vi "SaveJournalGen.vi"(7 "CheminSauv":path=path "C:/Données/Run003" caption="Fichier de Sauvegarde", 8 "error in":errorcluster, 10 "Include Date_Time":bool=TRUE, 11 "Journal Text":string) -> (0 "error out":errorcluster, 3 "chaîne de journal":string)   [LabVIEW 2019]
doc: "Ce Vi sauvegarde les données sous forme de collonnes dans le fichier texte de sauvegarde"
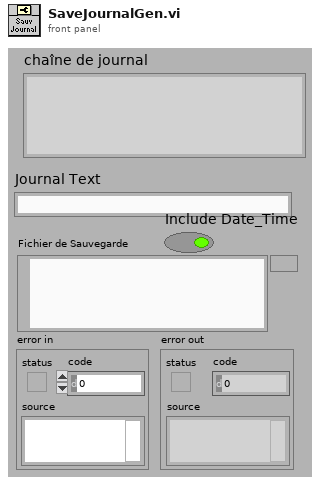
[diagram p1: front panel]
types:
  T1 = enum16{"open", "open or create", "create or replace", "create", "open (read only)"}
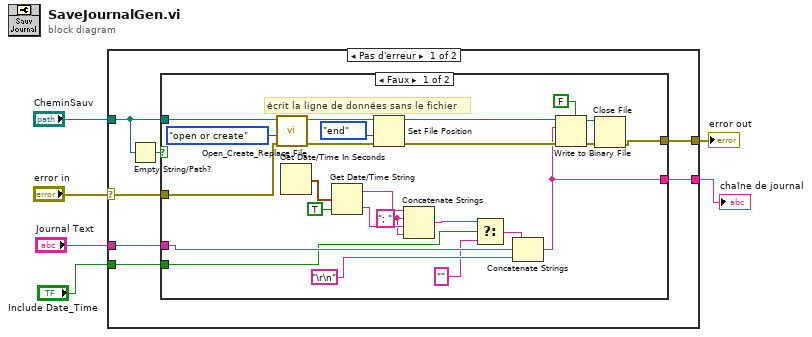
[diagram p0: block diagram]
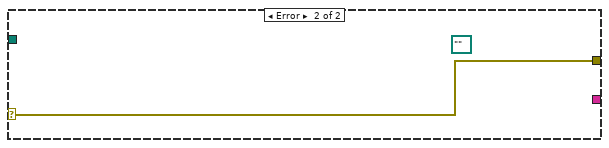
[diagram p3: hidden frame]
diagram:
  n1 = case shown="Pas d'erreur" "error in" {
    selector: "error in" -> [w12 w39]
    tunnel: [w13 w39] -> w6
    tunnel: "CheminSauv" -> [w10 _]
    tunnel: "Journal Text" -> [w9 _]
    tunnel: [w8 _] -> w2
    tunnel: "Include Date_Time" -> [w7 _]
    frame No Error {
      n2 = Empty String/Path?(string/path=w10) -> (empty?=w11:bool)
      n3 = case shown="Faux" w11 {
        tunnel: [w32 w38] -> w13
        tunnel: w12 -> [w31 w38]
        tunnel: w10 -> [w30 _]
        tunnel: w9 -> [w20 _]
        tunnel: [w16 _] -> w8
        tunnel: w7 -> [w14 _]
        frame False {
          w21 = "; " ("élément")
          # "écrit la ligne de données sans le fichier"
          n4 = call <vilib>:"Open_Create_Replace File.vi"("error in (no error)"=w31, "function (open:0)"=T1."open or create", "file path"=w30) -> ("error out"=w37:errorcluster, "refnum"=w33:refnum<file>)  [unwired: 5 in, 2 out]
          n5 = Get Date/Time In Seconds() -> (seconds since 1Jan1904=w23:timestamp)
          n6 = Get Date/Time String(seconds (now)=w23, want seconds? (F)=TRUE ("secondes ? (F)")) -> (date string=w25:string, time string=w22:string)  [unwired: 1 in]
          n7 = Set File Position(refnum=w33, from (0:start)=enum16{"start", "end", "current"}."end" ("pos mode (0:2)"), error in=w37) -> (refnum out=w28:refnum<file>, error out=w27:errorcluster)  [unwired: 1 in]
          n8 = Concatenate Strings(w25, w21, w22, w21) -> (w18:string)
          n9 = Select(t=w18, s=w14, f="" ("cas faux")) -> (s? t:f=w17:string)
          n10 = Concatenate Strings(w17, w20, "\r\n") -> (w16:string)
          n11 = Write to Binary File(file (use dialog)=w28, data=w16, error in=w27, 5:FALSE ("ajouter une taille de tableau ou de chaîne ? (V)")) -> (refnum out=w34:refnum<file>, error out=w36:errorcluster)  [unwired: 2 in, 1 out]
          n12 = Close File(refnum=w34, error in=w36) -> (error out=w32:errorcluster)  [unwired: 1 out]
        }
        frame True {
          # "path vide: on ne sauvegarde pas"
        }
      }
    }
    frame Error {
      (unwired) path "" ("path")
    }
  }
  "error out" <- w6
  "chaîne de journal" <- w2
